vi "decodeStream.vi"(8 "error in (no error)":errorcluster, 9 "beginIndex":i32, 10 "binary stream":u8[](array[numeric]), 11 "tBSONObjectID in":refnum<class "tBSONObjectID.lvclass">) -> (0 "error out":errorcluster, 1 "endIndex":i32, 2 "binary stream out":u8[](array[numeric]), 3 "tBSONObjectID out":refnum<class "tBSONObjectID.lvclass">)   [LabVIEW 2013, in "BSON.lvlib" / "tBSONObjectID.lvclass"]
uses:
  tBSONObjectID.lvclass
  tBSONElement/tBSONElement.lvclass
  status.ctl
  tBSONObjectID.lvclass/tBSONObjectID.ctl
  BSON.lvlib
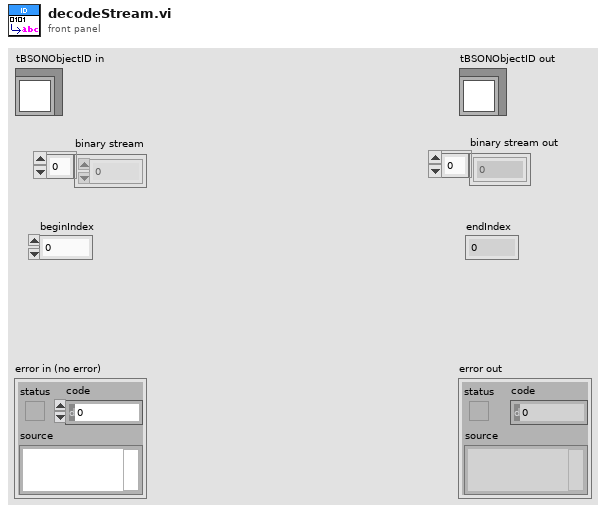
[diagram p1: front panel]
types:
  T1 = typedef "BSON.lvlib/status.ctl" = enum16{"Stream Corrupted or Ended Abruptly", "Incorrect Type In Stream", "ObjectID Invalid", "Method Not Implemented", "Invalid Name", "Invalid URI", "AutoReconnect", "Operation Failed", "Incorrectly Configured", "Cursor Not Found", "Timeout", "Invalid Type", "Empty Name", "Duplicate Name", "MD5Incorrect"}
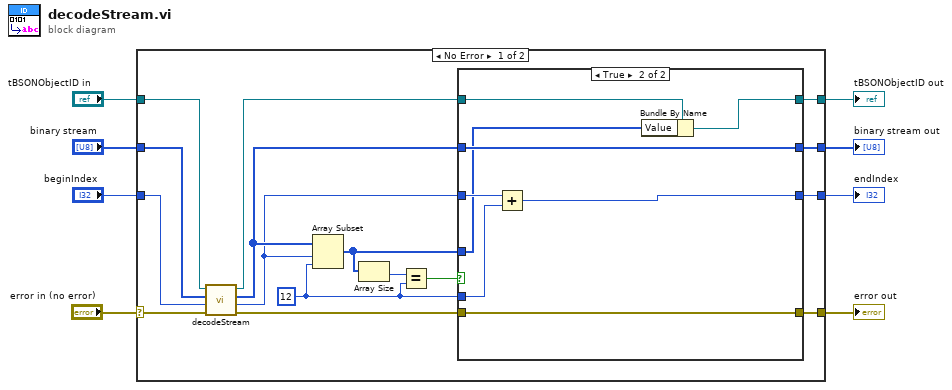
[diagram p0: block diagram]
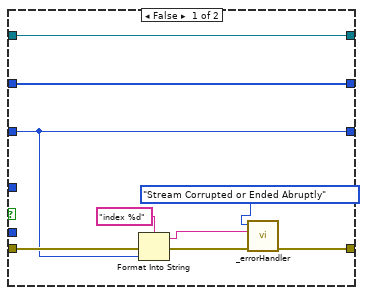
[diagram p2: hidden frame]
diagram:
  n1 = case shown="No Error" "error in (no error)" {
    selector: "error in (no error)" -> [w24 w42]
    tunnel: "beginIndex" -> [w21 w43]
    tunnel: "binary stream" -> [w22 w44]
    tunnel: "tBSONObjectID in" -> [w23 w45]
    tunnel: [w19 w45] -> w4
    tunnel: [w17 w44] -> w3
    tunnel: [w13 w43] -> w2
    tunnel: [w15 w42] -> w1
    frame No Error {
      w10 = 12
      n2 = call-parent "decodeStream.vi"("error in (no error)"=w24, "beginIndex"=w21, "binary stream"=w22, "tBSONElement in"=w23) -> ("error out"=w16:errorcluster, "endIndex"=w14:i32, "binary stream out"=w18:u8[], "tBSONElement out"=w20:refnum<class "tBSONObjectID.lvclass">)  [unwired: 4 in]
      n3 = Array Subset(array=w18, index=w14, length=w10) -> (w12:u8[])
      n4 = Array Size(array=w12) -> (size(s)=w11:i32)
      n5 = Equal?(x=w11, y=w10) -> (x = y?=w9:bool)
      n6 = case shown="True" w9 {
        tunnel: w20 -> [w33 w37]
        tunnel: [w33 w35] -> w19
        tunnel: w18 -> [w32 w41]
        tunnel: [w32 w41] -> w17
        tunnel: w16 -> [w27 w34]
        tunnel: [w26 w34] -> w15
        tunnel: w14 -> [w25 w40]
        tunnel: w10 -> [_ w39]
        tunnel: [w25 w38] -> w13
        tunnel: w12 -> [_ w36]
        frame False {
          n7 = Format Into String(format string="index %d", error in=w27, w25) -> (resulting string=w30:string, error out=w29:errorcluster)  [unwired: 1 in]
          n8 = call "_errorHandler.vi"("error in (no error)"=w29, "Additional Text"=w30, "Error Type"=status."Stream Corrupted or Ended Abruptly") -> ("error out"=w26:errorcluster)  [unwired: 8 in]
        }
        frame True {
          n9 = Add(x=w40, y=w39) -> (x+y=w38:i32)
          n10 = Bundle By Name(cluster=w37, "Value"=w36) -> (w35:refnum<class "tBSONObjectID.lvclass">)
        }
      }
    }
    frame Error {
    }
  }
  "error out" <- w1
  "tBSONObjectID out" <- w4
  "binary stream out" <- w3
  "endIndex" <- w2
